vi "DataLib.unpack description data.vi"(1 "serviceData":T1, 2 "descriptor":string, 5 "error in (no error)":errorcluster) -> (15 "header":string, 16 "DaqDevs":string[](array[string]), 17 "headerID":dbl, 19 "error out":errorcluster)   [LabVIEW 2014, in "DataLib.lvlib"]
doc: "This routine can be used to unpack the data received from the DIM service \"EVENTBUILDERNAME_dataDescription\"."
uses:
  DataLib.lvlib
  CS_Core/CSSystem/CoreDefs/CoreDefs.rawDataType.ctl
  CS_Core/CSSystem/CoreLib/CoreLib.lvlib
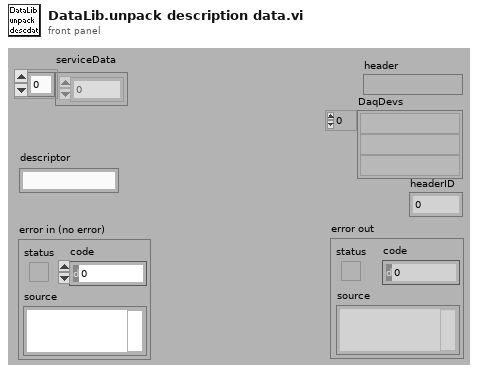
[diagram p1: front panel]
types:
  T1 = typedef "CoreDefs.rawDataType.ctl" = i8[]
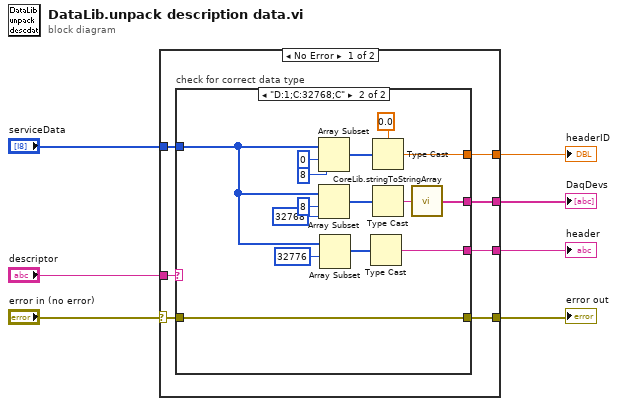
[diagram p0: block diagram]
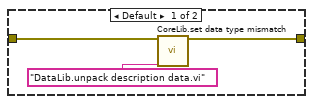
[diagram p2: hidden frame]
diagram:
  n1 = case shown="No Error" "error in (no error)" {
    selector: "error in (no error)" -> [w8 w33]
    tunnel: [w14 _] -> w7
    tunnel: [w13 _] -> w6
    tunnel: [w12 _] -> w5
    tunnel: "descriptor" -> [w11 _]
    tunnel: "serviceData" -> [w10 _]
    tunnel: [w9 w33] -> w2
    frame No Error {
      n2 = case "check for correct data type" shown="\"D:1;C:32768;C\"" w11 {
        tunnel: [_ w24] -> w14
        tunnel: [_ w23] -> w13
        tunnel: [_ w20] -> w12
        tunnel: w10 -> [_ w19]
        tunnel: [w17 w18] -> w9
        tunnel: w8 -> [w16 w18]
        frame Default {
          n3 = call "CoreLib.set data type mismatch.vi"("error in (no error)"=w16, "error source"="DataLib.unpack description data.vi") -> ("error out"=w17:errorcluster)  [unwired: 17 in]
        }
        frame "D:1;C:32768;C" {
          n4 = Array Subset(array=w19, index=0, length=8) -> (w30:T1)
          n5 = Array Subset(array=w19, index=8, length=32768) -> (w27:T1)
          n6 = Array Subset(array=w19, index=32776) -> (w25:T1)  [unwired: 1 in]
          n7 = Type Cast(x=w25) -> (*(type *) &x=w23:string)  [unwired: 1 in]
          n8 = Type Cast(type=0.0, x=w30) -> (*(type *) &x=w20:dbl)
          n9 = Type Cast(x=w27) -> (*(type *) &x=w22:string)  [unwired: 1 in]
          n10 = call "CoreLib.stringToStringArray.vi"("String"=w22) -> ("Array"=w24:string[])
        }
      }
    }
    frame Error {
    }
  }
  "header" <- w6
  "DaqDevs" <- w7
  "headerID" <- w5
  "error out" <- w2
